vi "Ctor.vi"(8 "error in (no error)":errorcluster, 10 "Password (None)":string, 11 "URL (Local Default)":string="ws://127.0.0.1:4455") -> (0 "error out":errorcluster, 3 "OBS out":refnum<class "OBS.lvclass">)   [LabVIEW 2022 SP3, in "obs-websocket-lv.lvlib" / "OBS.lvclass"]
uses:
  OBS.lvclass
  OBS.lvclass/OBS.ctl
  Response/Response.lvclass
  Client Message/Client Message.lvclass
  Client Message.ctl
  Command.ctl
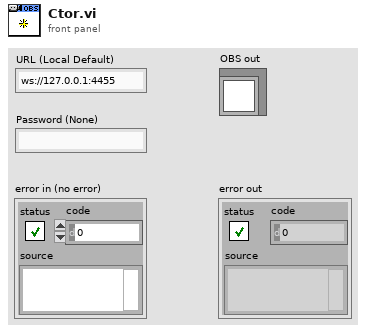
[diagram p1: front panel]
types:
  T1 = typedef "obs-websocket-lv.lvlib/OBS.lvclass/Command.ctl" = enum16{"Open", "Close", "Stop"}
  T2 = typedef "obs-websocket-lv.lvlib/OBS.lvclass/Client Message.ctl" = cluster{"Message":refnum<class "Client Message.lvclass">, "Response Notifier":refnum<notifier>}
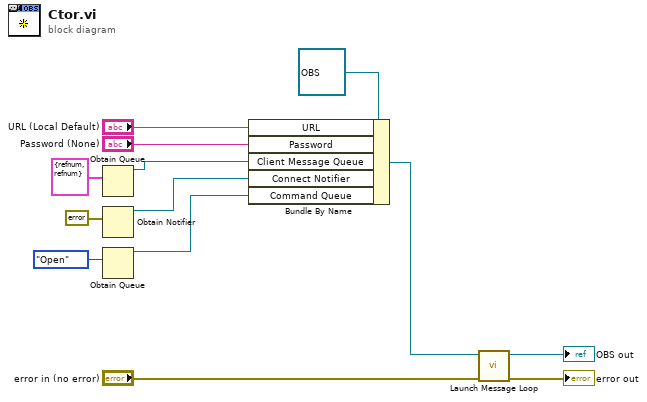
[diagram p0: block diagram]
diagram:
  n1 = Obtain Queue(element data type=T2 {"Message"=refnum, "Response Notifier"=refnum} ("Client Message")) -> (queue out=w11:refnum<queue>)  [unwired: 4 in, 2 out]
  n2 = Obtain Notifier(notification data type=errorcluster {"status"=FALSE, "code"=0, "source"=""} ("error constant")) -> (notifier out=w7:refnum<notifier>)  [unwired: 3 in, 2 out]
  n3 = Obtain Queue(element data type=Command."Open" ("Command")) -> (queue out=w5:refnum<queue>)  [unwired: 4 in, 2 out]
  n4 = Bundle By Name(cluster=refnum<class "OBS.lvclass"> refnum ("OBS in"), "URL"="URL (Local Default)", "Password"="Password (None)", "Client Message Queue"=w11, "Connect Notifier"=w7, "Command Queue"=w5) -> (w4:refnum<class "OBS.lvclass">)
  n5 = call "Launch Message Loop.vi"("error in (no error)"="error in (no error)", "OBS in"=w4) -> ("error out"=→"error out":errorcluster, "OBS out"=→"OBS out":refnum<class "OBS.lvclass">)  [unwired: 8 in]
